vi "Advance past colon.vi"(7 "JSON":string, 9 "Offset":i32, 11 "State":T1=enum."Leading Whitespace") -> (1 "index":i32, 3 "State":T1=enum."Value end")   [LabVIEW 2024, in "JSONtext.lvlib"]
uses:
  JSONtext.lvlib
  Parsing State.ctl
  Advance past Line Ending.vi
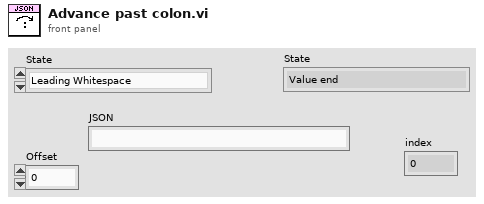
[diagram p1: front panel]
types:
  T1 = typedef "JSONtext.lvlib/Parsing State.ctl" = enum16{"Parser Error", "Object", "Array", "String", "Number/Other", "Leading Whitespace", "Object end", "Array end", "Value end"}
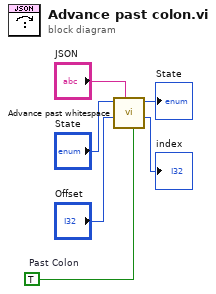
[diagram p0: block diagram]
diagram:
  w1 = TRUE  # Past Colon
  n1 = call "Advance past whitespace.vi"("Past Colon"=w1, "JSON"="JSON", "Offset"="Offset", "Parser State in"="State") -> ("Offset of first non-whitespace"=→"index":i32, "Parser State"=→"State":T1)  [unwired: 5 in, 1 out]
